vi "Example Plant Dynamics.vi"(11 "Motor Velocity Command (deg/s)":dbl) -> (0 "Motor Velocity (deg/s)":dbl, 3 "Force":dbl)   [LabVIEW 2018]
uses:
  <vilib>/ptbypt/NI_PtbyPt.lvlib
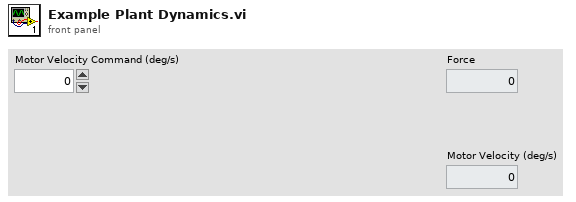
[diagram p1: front panel]
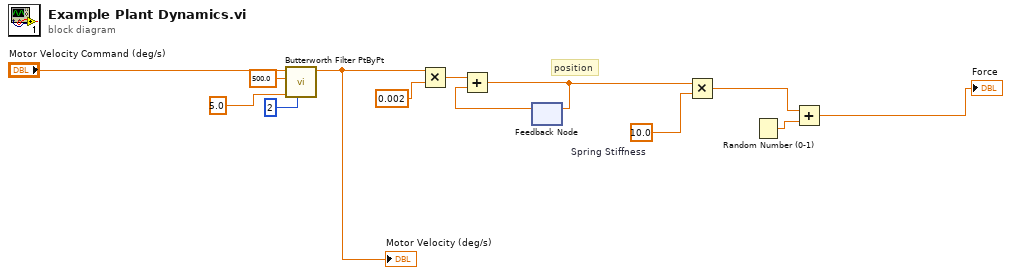
[diagram p0: block diagram]
diagram:
  w5 = 10.0  # Spring Stiffness
  # "position"
  n1 = call <vilib>:"Butterworth Filter PtByPt.vi"("order"=2, "low cutoff freq: fl"=5.0, "sampling freq: fs"=500.0, "x"="Motor Velocity Command (deg/s)") -> ("Filtered x"=w4:dbl)  [unwired: 5 in, 1 out]
  "Motor Velocity (deg/s)" <- w4
  n2 = Multiply(x=w4, y=0.002) -> (x*y=w8:dbl)
  n3 = feedback #1() -> (w7:dbl)  [unwired: 1 in]
  n4 = Add(x=w8, y=w7) -> (x+y=w6:dbl)
  n5 = feedback-in #1(w6) -> ()
  n6 = Multiply(x=w6, y=w5) -> (x*y=w2:dbl)
  n7 = Random Number (0-1)() -> (number: 0 to 1=w3:dbl)
  n8 = Add(x=w2, y=w3) -> (x+y=→"Force":dbl)
